vi "Measurement Logic.vi"() -> ()   [LabVIEW 2020, in "NIDmmMeasurement.lvlib"]
uses:
  NIDmmMeasurement.lvlib
  <vilib>/MeasurementLink/MeasurementLink Session Management/Session Reservation/Session Reservation.lvclass
  Measurement Results.ctl
  <instrlib>/niDMM/nidmm.llb/niDMM Configure Measurement Digits.vi
  <instrlib>/niDMM/nidmm.llb/niDMM Resolution in Digits.ctl
  <vilib>/MeasurementLink/MeasurementLink niDMM/MeasurementLink niDMM.lvlib
  <vilib>/MeasurementLink/MeasurementLink niDMM/Initialize Sessions - 1Sess.vi
  <vilib>/MeasurementLink/MeasurementLink Measurement Server/Measure Call Context/Measure Call Context.lvclass
  Measurement Configuration.ctl
  ResolutionInDigits.ctl
panel:
  out "Measurement Context out":refnum<class "Measure Call Context.lvclass">
  in  "Measurement Context":refnum<class "Measure Call Context.lvclass">
  out "Measurement Results":T1 {"Absolute Resolution" format="%#_3p"; "Measurement" format="%.6p"}
  in  "Measurement Configuration":T2={"pin_name"="", "Range"=10.0, "Measurement Type"=enum."DC Volts", "Resolution in Digits"=enum."5 1/2"} {"Range" format="%.2f"}
  out "error out":errorcluster
  in  "error in":errorcluster
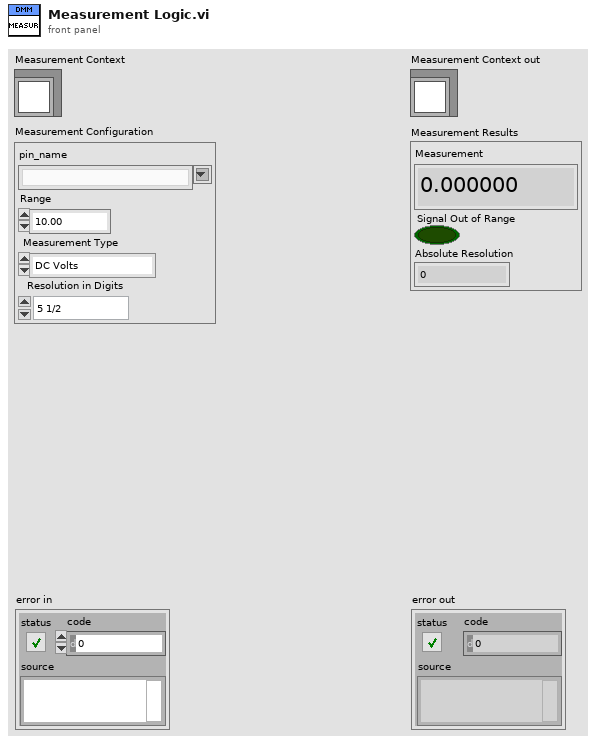
[diagram p1: front panel]
types:
  T1 = typedef "NIDmmMeasurement.lvlib/Measurement Results.ctl" = cluster{"Measurement":dbl, "Signal Out of Range":bool, "Absolute Resolution":dbl}
  T2 = typedef "NIDmmMeasurement.lvlib/Measurement Configuration.ctl" = cluster{"pin_name":string, "Range":dbl, "Measurement Type":enum32{"DC Volts", "AC Volts", "DC Current", "AC Current", "2-wire Resistance", "4-wire Resistance", "Diode", "Frequency", "Period", "AC Volts DC Coupled", "Capacitance", "Inductance", "Temperature"}, "Resolution in Digits":T3}
  T3 = typedef "NIDmmMeasurement.lvlib/ResolutionInDigits.ctl" = enum32{"3 1/2", "4 1/2", "5 1/2", "6 1/2", "7 1/2"}
  T4 = enum32{"DC Volts", "AC Volts", "DC Current", "AC Current", "2-wire Resistance", "4-wire Resistance", "Diode", "Frequency", "Period", "AC Volts DC Coupled", "Capacitance", "Inductance", "Temperature"}
  T5 = typedef "niDMM Resolution in Digits.ctl" = dbl
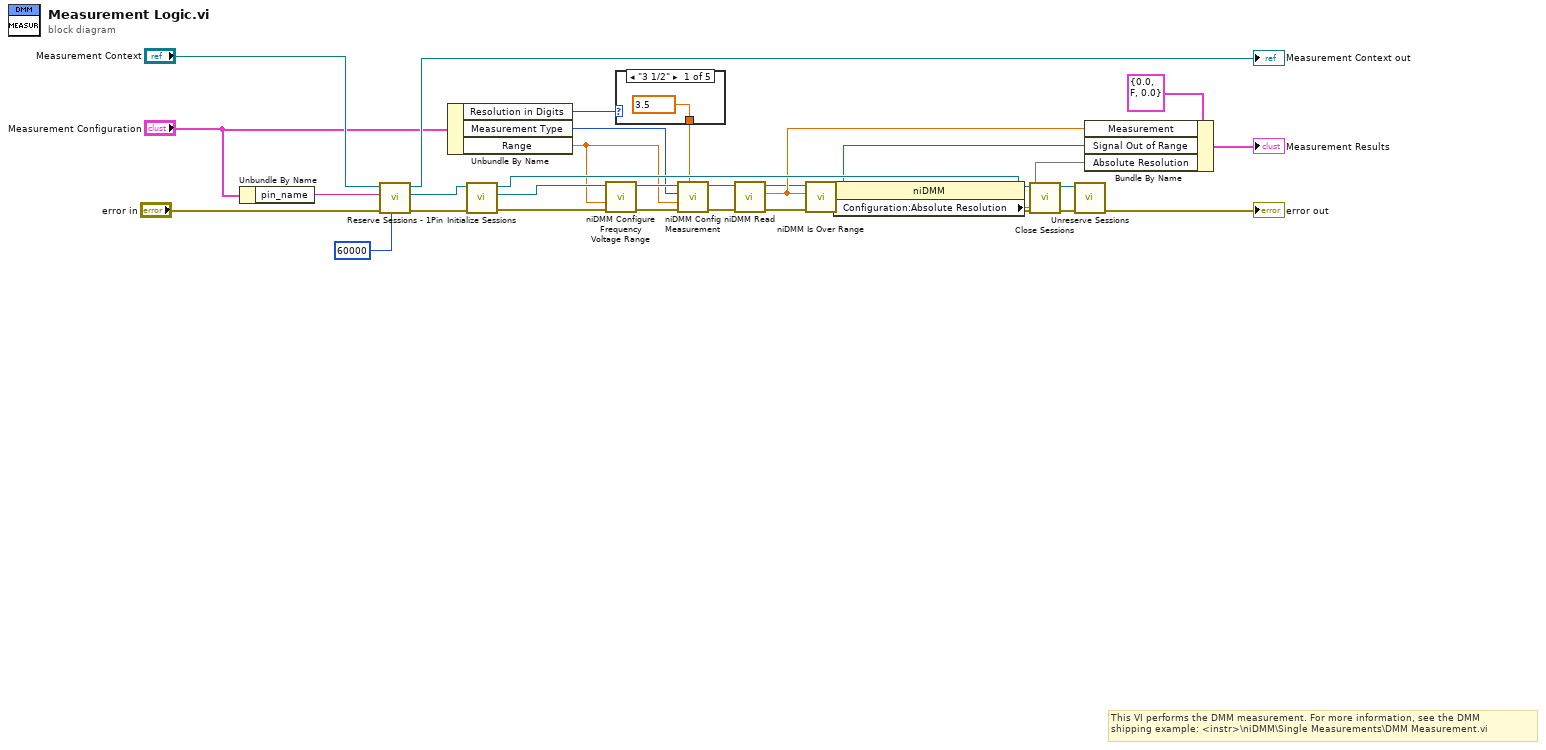
[diagram p0: block diagram]
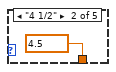
[diagram p2: hidden frame]
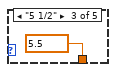
[diagram p3: hidden frame]
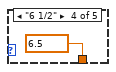
[diagram p4: hidden frame]
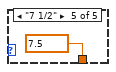
[diagram p5: hidden frame]
diagram:
  # "This VI performs the DMM measurement. For more information, see the DMM\nshipping example: <instr>\\niDMM\\Single Measurements\\DMM Measurement.vi"
  n1 = Unbundle By Name("Measurement Configuration") -> ("pin_name"=w32:string)
  n2 = call <vilib>:"Reserve Sessions - 1Pin.vi"("timeout (ms)"=60000, "error in"="error in", "pin or relay name"=w32, "measurement context in"="Measurement Context") -> ("error out"=w28:errorcluster, "session reservation out"=w29:refnum<class "Session Reservation.lvclass">, "measurement context out"=→"Measurement Context out":refnum<class "Measure Call Context.lvclass">)  [unwired: 5 in]
  n3 = Unbundle By Name("Measurement Configuration") -> ("Resolution in Digits"=w2:T3, "Measurement Type"=w4:T4, "Range"=w5:dbl)
  n4 = call-poly <vilib>:"Initialize Sessions.vi"("error in"=w28, "session reservation in"=w29) -> ("error out"=w9:errorcluster, "session"=w8:refnum<k15>, "session reservation out"=w24:refnum<class "Session Reservation.lvclass">)  [unwired: 6 in, 1 out]
  n5 = call <instrlib>:"niDMM Configure Frequency Voltage Range.vi"("Frequency Voltage Range"=w5, "error in (no error)"=w9, "instrument handle"=w8) -> ("error out"=w17:errorcluster, "instrument handle out"=w16:refnum<k15>)  [unwired: 7 in]
  n6 = case shown="\"3 1/2\"" w2 {
    tunnel: [w33 w34 w35 w36 w37] -> w1
    frame "3 1/2" {
      w33 = T5 3.5 items=["3 1/2"=3.5, "4 1/2"=4.5, "5 1/2"=5.5, "6 1/2"=6.5, "7 1/2"=7.5] ("Resolution in Digits")
    }
    frame "4 1/2" {
      w34 = T5 4.5 items=["3 1/2"=3.5, "4 1/2"=4.5, "5 1/2"=5.5, "6 1/2"=6.5, "7 1/2"=7.5] ("Resolution in Digits")
    }
    frame "5 1/2" {
      w35 = T5 5.5 items=["3 1/2"=3.5, "4 1/2"=4.5, "5 1/2"=5.5, "6 1/2"=6.5, "7 1/2"=7.5] ("Resolution in Digits")
    }
    frame "6 1/2" {
      w36 = T5 6.5 items=["3 1/2"=3.5, "4 1/2"=4.5, "5 1/2"=5.5, "6 1/2"=6.5, "7 1/2"=7.5] ("Resolution in Digits")
    }
    frame "7 1/2" {
      w37 = T5 7.5 items=["3 1/2"=3.5, "4 1/2"=4.5, "5 1/2"=5.5, "6 1/2"=6.5, "7 1/2"=7.5] ("Resolution in Digits")
    }
  }
  n7 = call-poly <instrlib>:"niDMM Config Measurement.vi"("Range"=w5, "Resolution in Digits"=w1, "error in (no error)"=w17, "Function"=w4, "instrument handle"=w16) -> ("error out"=w12:errorcluster, "instrument handle out"=w13:refnum<k15>)  [unwired: 5 in]
  n8 = call <instrlib>:"niDMM Read.vi"("error in (no error)"=w12, "instrument handle"=w13) -> ("error out"=w19:errorcluster, "Measurement"=w22:dbl, "instrument handle out"=w14:refnum<k15>)  [unwired: 7 in]
  n9 = call <instrlib>:"niDMM Is Over Range.vi"("error in (no error)"=w19, "Measurement"=w22, "instrument handle"=w14) -> ("error out"=w18:errorcluster, "Over Range?"=w21:bool, "instrument handle out"=w15:refnum<k15>)  [unwired: 6 in]
  n10 = property class="niDMM"(reference=w15, error in=w18) -> (error out=w6:errorcluster, "Configuration:Absolute Resolution"=w20)  [unwired: 1 out]
  n11 = call <vilib>:"Close Sessions.vi"("error in"=w6, "session reservation in"=w24) -> ("error out"=w27:errorcluster, "session reservation out"=w26:refnum<class "Session Reservation.lvclass">)  [unwired: 8 in]
  n12 = call <vilib>:"Unreserve Sessions.vi"("error in"=w27, "session reservation in"=w26) -> ("error out"=→"error out":errorcluster)  [unwired: 9 in]
  n13 = Bundle By Name(cluster=T1 {"Measurement"=0.0, "Signal Out of Range"=FALSE, "Absolute Resolution"=0.0} ("Measurement Results"), "Measurement"=w22, "Signal Out of Range"=w21, "Absolute Resolution"=w20) -> (→"Measurement Results":T1)
